vi "N-Double FFT Mesurament (Control - Init Wave&Window - Snapshot - DoubleFFT - Latency - Low Freq) RT Test.vi"() -> ()   [LabVIEW 2014]
uses:
  <vilib>/rvi/interface/nirviOpenFPGA/nirviOpenFPGA.xnode
  <vilib>/rvi/interface/nirviMethod/nirviMethod.xnode
  <vilib>/FPGAPlugInAG/Dynamic/niLvFpga_ConfigureFifo_Dynamic.vi
  <vilib>/rvi/errors/niLvFpgaMergeErrorWithErrorCode.vi
  <vilib>/FPGAPlugInAG/Dynamic/niLvFpga_StartFifo_Dynamic.vi
  <vilib>/FPGAPlugInAG/Dynamic/niLvFpga_Run_Dynamic.vi
  <vilib>/FPGAPlugInAG/Dynamic/niLvFpga_Abort_Dynamic.vi
  <vilib>/rvi/interface/nirviCloseFPGA/nirviCloseFPGA.xnode
  <vilib>/rvi/interface/nirviReadWriteControl/nirviReadWriteControl.xnode
  <vilib>/rvi/interface/Simulation/niFpgaSimulationCallBeginRW.vi
  <vilib>/rvi/errors/niLvFpgaAdjustHostInterfaceError.vi
  <vilib>/FPGAPlugInAG/Dynamic/niLvFpga_ReadFifo_Dynamic.vi
  <vilib>/Platform/TimedLoop/XDataNode/XDataNode.xnode
  <vilib>/Platform/TimedLoop/XDataNode/nitl_modes.ctl
  <vilib>/Platform/TimedLoop/XDataNode/XDNodeRunTimeDep.lvlib
  <vilib>/Platform/TimedLoop/XDataNode/wakeup.ctl
  <vilib>/Platform/TimedLoop/XDataNode/timing_clust.ctl
  <vilib>/FPGAPlugInAG/Dynamic/niLvFpga_Reset_Dynamic.vi
  NiFpgaLv.dll
  <vilib>/Utility/error.llb/Error Cluster From Error Code.vi
  FPGA Target/Test VIs/Double FFT Mesurament (Control - Init Wave&Window - Snapshot - DoubleFFT - Latency - Low Freq - PARAM LEO) test.vi
  <vilib>/FPGAPlugInAG/Dynamic/niLvFpga_Close_Dynamic.vi
panel:
  out "N-FFT":dbl[](graph)
  out "Write memory complete":bool
  in  "#Signals":u32=1
  in  "stop":bool
  in  "Initial Latency points":u32(slide)=10 scale=0.0..1249.0
  out "Elements Remaining FFT":u32
  out "Elements Remaining Signal":u32
  out "N-Signals":dbl[](graph)
  in  "Snapshot":bool
  in  "Windowing":T1(ring)
  in  "first bin":i32=15
  in  "last bin":i32=255
  in  "lower limit 2":u32(slide)=725 scale=625.0..738.0
  in  "lower limit 1":u32(slide)=100 scale=0.0..113.0
  # "WARNING:\nOnce pressed wait untill the end of operation"
  # "OFFLINE parameters"
  # "Max Detection FFT bin range"
  # "TEST"
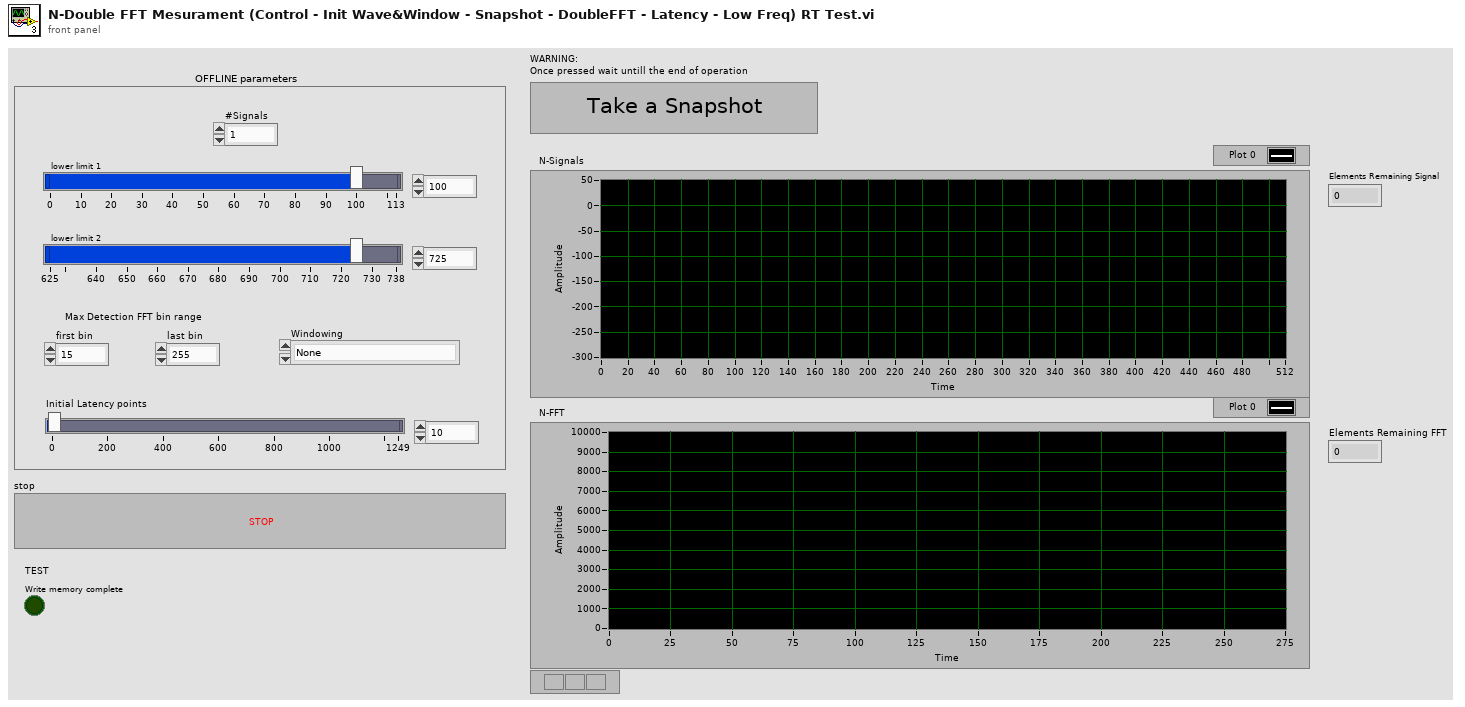
[diagram p1: front panel]
types:
  T1 = enum16{"None", "Hanning", "Hamming", "Blackman", "Blackman-Harris"}
  T2 = typedef "XDNodeRunTimeDep.lvlib/timing_clust.ctl" = cluster{"Expected End [f-1]":u64, "Actual End [f-1]":u64, "Finished Late? [f-1]":bool, "Expected End [i-1]":u64, "Actual End [i-1]":u64, "Finished Late? [i-1]":bool, "Expected Start [i]":u64, "Actual Start [i]":u64, "Expected Start [f]":u64, "Actual Start [f]":u64, "Source Name":string, "Structure Name":string, "Period":i64, "Deadline":i64, "Offset":i64, "Start":i64, "Priority":i32, "Timeout":i32, "Mode":T3, "Wakeup Reason":T4, "Error":errorcluster, "Source Type":string, "Secondary Source Type":string, "Global End Time":u64, "Global Start Time":u64, "Frame Duration":u64, "Iteration Duration":u64, "Assigned CPU":i32, "I/O Scan Engine Mode":u32}
  T3 = typedef "XDNodeRunTimeDep.lvlib/nitl_modes.ctl" = enum32{"No Change", "Process missed periods, maintain original phase", "Discard missed periods, maintain original phase", "Process missed periods, ignore original phase", "Discard missed periods, ignore original phase"}
  T4 = typedef "XDNodeRunTimeDep.lvlib/wakeup.ctl" = enum32{"Normal", "Aborted", "Asynchronous wakeup", "Timing source error", "Timed loop error", "Timeout"}
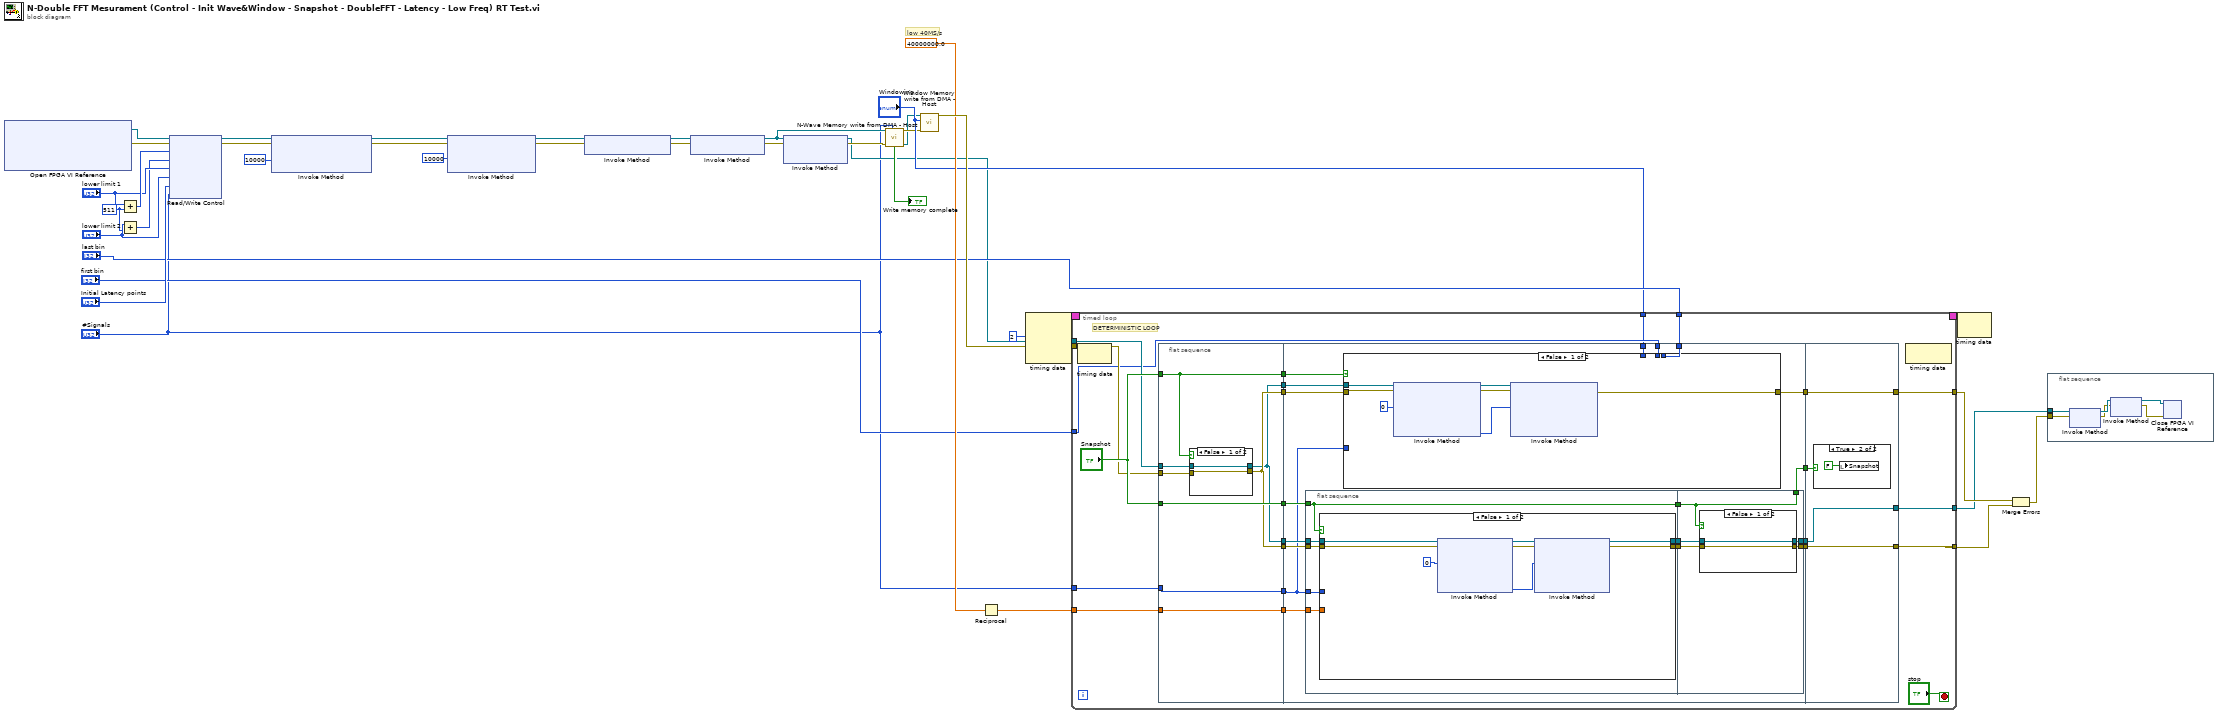
[diagram p0: block diagram]
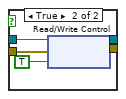
[diagram p2: hidden frame]
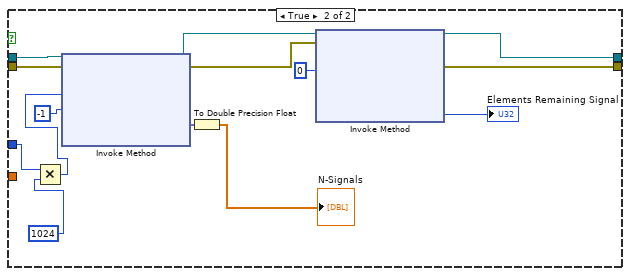
[diagram p3: hidden frame]
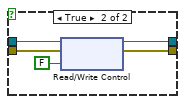
[diagram p4: hidden frame]
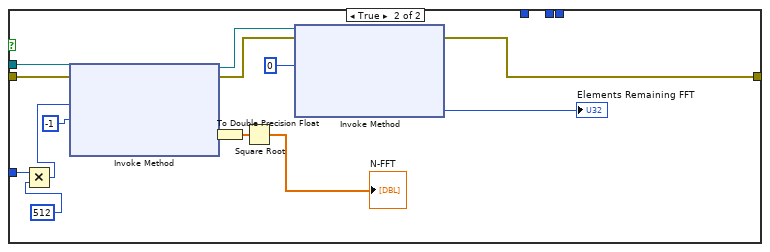
[diagram p5: hidden frame]
diagram:
  w35 = u32 511 ("y")
  # "low 40MS/s"
  n1 = xnode "Open FPGA VI Reference"() -> ("FPGA VI Reference Out"=w34:refnum<k20>, "error out"=w33:errorcluster)  [unwired: 2 in]
  n2 = Add(x="lower limit 1", y=w35) -> (x+y=w39:u32)
  n3 = Add(x="lower limit 2", y=w35) -> (x+y=w37:u32)
  n4 = xnode "Read/Write Control"("FPGA VI Reference In"=w34, "error in"=w33, "upper limit 1"=w39, "upper limit 2"=w37, "lower limit 1"="lower limit 1", "lower limit 2"="lower limit 2", "Latency points"="Initial Latency points", "n"="#Signals") -> ("FPGA VI Reference Out"=w31:refnum<k20>, "error out"=w30:errorcluster)
  n5 = xnode "Invoke Method"("FPGA VI Reference In"=w31, "error in"=w30, "Requested Depth"=u32 10000) -> ("FPGA VI Reference Out"=w11:refnum<k20>, "error out"=w12:errorcluster)  [unwired: 1 out]
  n6 = xnode "Invoke Method"("FPGA VI Reference In"=w11, "error in"=w12, "Requested Depth"=u32 10000) -> ("FPGA VI Reference Out"=w23:refnum<k20>, "error out"=w24:errorcluster)  [unwired: 1 out]
  n7 = xnode "Invoke Method"("FPGA VI Reference In"=w23, "error in"=w24) -> ("FPGA VI Reference Out"=w9:refnum<k20>, "error out"=w10:errorcluster)
  n8 = xnode "Invoke Method"("FPGA VI Reference In"=w9, "error in"=w10) -> ("FPGA VI Reference Out"=w2:refnum<k20>, "error out"=w22:errorcluster)
  n9 = xnode "Invoke Method"("FPGA VI Reference In"=w2, "error in"=w22) -> ("FPGA VI Reference Out"=w3:refnum<k20>, "error out"=w7:errorcluster)  [unwired: 1 in]
  n10 = call "N-Wave Memory write from DMA - Host.vi"("n"="#Signals", "error in"=w7, "FPGA VI Reference In"=w2) -> ("FPGA VI Reference Out"=w5:refnum<k20>, "error out"=w6:errorcluster, "Write memory complete"=→"Write memory complete":bool)  [unwired: 6 in]
  n11 = call "Window Memory write from DMA - Host.vi"("error in"=w6, "Enum"="Windowing", "FPGA VI Reference In"=w5) -> ("error out"=w32:errorcluster)  [unwired: 5 in, 3 out]
  n12 = Reciprocal(x=40000000.0 ("Sample Rate (S/s)")) -> (1/x=w26:dbl)
  n13 = node-c288(i64 2 ("Period")) -> (w21:T2)  [unwired: 3 in]
  n14 = timed-loop {
    tunnel: w3 -> [w58]
    tunnel: w32 -> [w59]
    tunnel: [w61] -> w18
    tunnel: w26 -> [w63]
    tunnel: [w62] -> w17
    timing: w21 -> [_]
    timing-out: [_] -> w20
    tunnel: "first bin" -> [w47]
    tunnel: "last bin" -> [w46]
    tunnel: [w44] -> w13
    tunnel: "Windowing" -> [w42]
    tunnel: "#Signals" -> [w40]
    stop <- "stop" stop-if-true
    # "DETERMINISTIC LOOP"
    n15 = node-c288() -> ()  [unwired: 1 in, 1 out]
    n16 = flat-sequence {
      tunnel: w58 -> [w69]
      tunnel: w59 -> [w70]
      tunnel: "Snapshot" -> [w67]
      tunnel: "Snapshot" -> [w72]
      tunnel: w63 -> [w73]
      tunnel: [w71] -> w57
      tunnel: [w73] -> w56
      tunnel: [w72] -> w55
      tunnel: [w67] -> w54
      tunnel: [w71] -> w53
      tunnel: [w68] -> w52
      tunnel: [w68] -> w51
      tunnel: [w66] -> w41
      tunnel: w40 -> [w66]
      tunnel: w57 -> [w94]
      tunnel: w56 -> [w93]
      tunnel: w55 -> [w87]
      tunnel: w54 -> [w90]
      tunnel: w53 -> [w89]
      tunnel: w52 -> [w88]
      tunnel: w51 -> [w95]
      tunnel: [w92] -> w50
      tunnel: [w91] -> w49
      tunnel: [w86] -> w48
      tunnel: w47 -> [w85]
      tunnel: w46 -> [w84]
      tunnel: [w83] -> w43
      tunnel: w42 -> [w82]
      tunnel: w41 -> [w81]
      tunnel: [w163] -> w61
      tunnel: [w164] -> w62
      tunnel: w50 -> [w164]
      tunnel: w49 -> [w163]
      tunnel: w48 -> [w162]
      tunnel: [w161] -> w44
      tunnel: w43 -> [w161]
      frame #0 {
        n17 = case shown="False" w67 {
          tunnel: [w74 w79] -> w71
          tunnel: w70 -> [w74 w78]
          tunnel: w69 -> [w75 w77]
          tunnel: [w75 w76] -> w68
          frame False {
          }
          frame True {
            n18 = xnode "Read/Write Control"("FPGA VI Reference In"=w77, "error in"=w78, "snapshot"=TRUE) -> ("FPGA VI Reference Out"=w76:refnum<k20>, "error out"=w79:errorcluster)
          }
        }
      }
      frame #1 {
        n19 = flat-sequence {
          tunnel: w95 -> [w105]
          tunnel: w94 -> [w104]
          tunnel: w93 -> [w103]
          tunnel: w87 -> [w100]
          tunnel: [w102] -> w98
          tunnel: [w101] -> w97
          tunnel: [w100] -> w96
          tunnel: w81 -> [w99]
          tunnel: [w130] -> w91
          tunnel: w98 -> [w132]
          tunnel: w97 -> [w131]
          tunnel: w96 -> [w129]
          tunnel: [w129] -> w86
          tunnel: [w128] -> w83
          frame #0 {
            n20 = case shown="False" w100 {
              tunnel: w105 -> [w112 w127]
              tunnel: w104 -> [w110 w126]
              tunnel: [w109 w120] -> w101
              tunnel: w103 -> [_ _]
              tunnel: [w106 w119] -> w102
              tunnel: w99 -> [_ w116]
              frame False {
                n21 = xnode "Invoke Method"("FPGA VI Reference In"=w112, "error in"=w110, "Number of Elements"=u32 0) -> ("FPGA VI Reference Out"=w108:refnum<k20>, "error out"=w107:errorcluster, "Elements Remaining"=w111:u32)  [unwired: 1 in, 1 out]
                n22 = xnode "Invoke Method"("FPGA VI Reference In"=w108, "error in"=w107, "Number of Elements"=w111) -> ("FPGA VI Reference Out"=w106:refnum<k20>, "error out"=w109:errorcluster)  [unwired: 1 in, 2 out]
              }
              frame True {
                n23 = Multiply(x=w116, y=u32 1024 ("Number of Elements")) -> (x*y=w117:u32)
                n24 = xnode "Invoke Method"("FPGA VI Reference In"=w127, "error in"=w126, "Number of Elements"=w117, "Timeout (ms)"=-1) -> ("FPGA VI Reference Out"=w122:refnum<k20>, "error out"=w121:errorcluster, "Data"=w124:fxp<+/-,12,12>[])  [unwired: 1 out]
                n25 = To Double Precision Float(number=w124) -> (double precision float=→"N-Signals":dbl[])
                n26 = xnode "Invoke Method"("FPGA VI Reference In"=w122, "error in"=w121, "Number of Elements"=u32 0) -> ("FPGA VI Reference Out"=w119:refnum<k20>, "error out"=w120:errorcluster, "Elements Remaining"=→"Elements Remaining Signal":u32)  [unwired: 1 in, 1 out]
              }
            }
          }
          frame #1 {
            n27 = case shown="False" w129 {
              tunnel: [w134 w137] -> w130
              tunnel: w132 -> [w133 w138]
              tunnel: w131 -> [w134 w136]
              tunnel: [w133 w135] -> w128
              frame False {
              }
              frame True {
                n28 = xnode "Read/Write Control"("FPGA VI Reference In"=w138, "error in"=w136, "snapshot"=FALSE) -> ("FPGA VI Reference Out"=w135:refnum<k20>, "error out"=w137:errorcluster)
              }
            }
          }
        }
        n29 = case shown="False" w90 {
          tunnel: w88 -> [w145 w156]
          tunnel: w89 -> [w142 w157]
          tunnel: [w141 w155] -> w92
          tunnel: w85 -> [_ _]
          tunnel: w84 -> [_ _]
          tunnel: w82 -> [_ _]
          tunnel: w81 -> [_ w148]
          frame False {
            n30 = xnode "Invoke Method"("FPGA VI Reference In"=w145, "error in"=w142, "Number of Elements"=u32 0) -> ("FPGA VI Reference Out"=w143:refnum<k20>, "error out"=w140:errorcluster, "Elements Remaining"=w144:u32)  [unwired: 1 in, 1 out]
            n31 = xnode "Invoke Method"("FPGA VI Reference In"=w143, "error in"=w140, "Number of Elements"=w144) -> ("error out"=w141:errorcluster)  [unwired: 1 in, 3 out]
          }
          frame True {
            n32 = Multiply(x=w148, y=u32 512 ("Number of Elements")) -> (x*y=w149:u32)
            n33 = xnode "Invoke Method"("FPGA VI Reference In"=w156, "error in"=w157, "Number of Elements"=w149, "Timeout (ms)"=-1) -> ("FPGA VI Reference Out"=w153:refnum<k20>, "error out"=w154:errorcluster, "Data"=w159:fxp<+,44,44>[])  [unwired: 1 out]
            n34 = To Double Precision Float(number=w159) -> (double precision float=w158:dbl[])
            n35 = Square Root(x=w158) -> (sqrt(x)=→"N-FFT":dbl[])
            n36 = xnode "Invoke Method"("FPGA VI Reference In"=w153, "error in"=w154, "Number of Elements"=u32 0) -> ("error out"=w155:errorcluster, "Elements Remaining"=→"Elements Remaining FFT":u32)  [unwired: 1 in, 2 out]
          }
        }
      }
      frame #2 {
        n37 = case shown="True" w162 {
          frame False {
          }
          frame True {
            n38 = local write "Snapshot"(FALSE ("Snapshot")) -> ()
          }
        }
      }
    }
    n39 = node-c288() -> ()  [unwired: 1 in, 1 out]
  }
  n40 = node-c288(w20) -> ()  [unwired: 1 out]
  n41 = Merge Errors(w17, w18) -> (w27:errorcluster)
  n42 = flat-sequence {
    tunnel: w27 -> [w171]
    tunnel: w13 -> [w166]
    frame #0 {
      n43 = xnode "Invoke Method"("FPGA VI Reference In"=w166, "error in"=w171) -> ("FPGA VI Reference Out"=w168:refnum<k20>, "error out"=w167:errorcluster)
      n44 = xnode "Invoke Method"("FPGA VI Reference In"=w168, "error in"=w167) -> ("FPGA VI Reference Out"=w169:refnum<k20>, "error out"=w170:errorcluster)
      n45 = xnode "Close FPGA VI Reference"("FPGA VI Reference In"=w169, "error in"=w170) -> ()  [unwired: 1 out]
    }
  }
